vi "Write Path Configuration.vi"(8 "error in (no error)":errorcluster, 9 "Value":path, 10 "Name":string, 11 "database-configuration in":refnum<class "configuration-database.lvclass">) -> (0 "error out":errorcluster, 3 "database-configuration out":refnum<class "configuration-database.lvclass">)   [LabVIEW 2020, in "configuration-database.lvlib" / "configuration-database.lvclass"]
uses:
  configuration-database.lvclass
  configuration-database.lvclass/configuration-database.ctl
  d7598d41-e364-4b12-88e5-b1ff7f28b338.vi
  <vilib>/Utility/error.llb/Error Cluster From Error Code.vi
  IConfigDBQueries/IConfigurationDatabaseQueries.lvclass
  externals/database-interface/IDatabase/IDatabase/IDatabase.lvclass
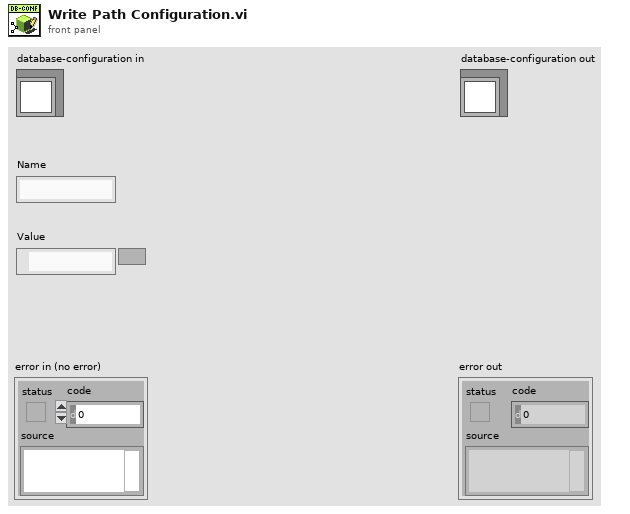
[diagram p1: front panel]
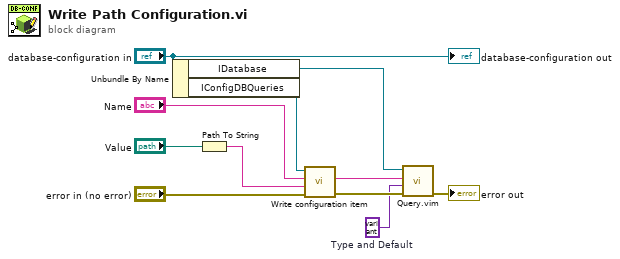
[diagram p0: block diagram]
diagram:
  w1 = variant  # Type and Default
  n1 = Unbundle By Name("database-configuration in") -> ("IDatabase"=w8:refnum<class "IDatabase.lvclass">, "IConfigDBQueries"=w9:refnum<class "IConfigurationDatabaseQueries.lvclass">)
  n2 = Path To String(path="Value") -> (string=w3:string)
  n3 = call-dynamic "Write configuration item.vi"("error in (no error)"="error in (no error)", "Value"=w3, "Name in"="Name", "IConfigDBQueries in"=w9) -> ("error out"=w10:errorcluster, "Query"=w11:string)  [unwired: 6 in]
  n4 = call "Query.vim"("error in (no error)"=w10, "Type and Default"=w1, "Query string"=w11, "IDatabase in"=w8) -> ("error out"=→"error out":errorcluster)  [unwired: 5 in, 2 out]
  "database-configuration out" <- "database-configuration in"
